vi "FindGit.vi"(8 "error in (no error)":errorcluster) -> (0 "error out":errorcluster, 2 "User Cancelled":bool, 3 "Git String":string)   [LabVIEW 2013]
uses:
  <vilib>/Utility/sysdir.llb/System Directory Type.ctl
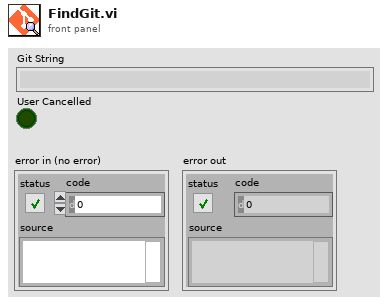
[diagram p1: front panel]
types:
  T1 = typedef "System Directory Type.ctl" = i32
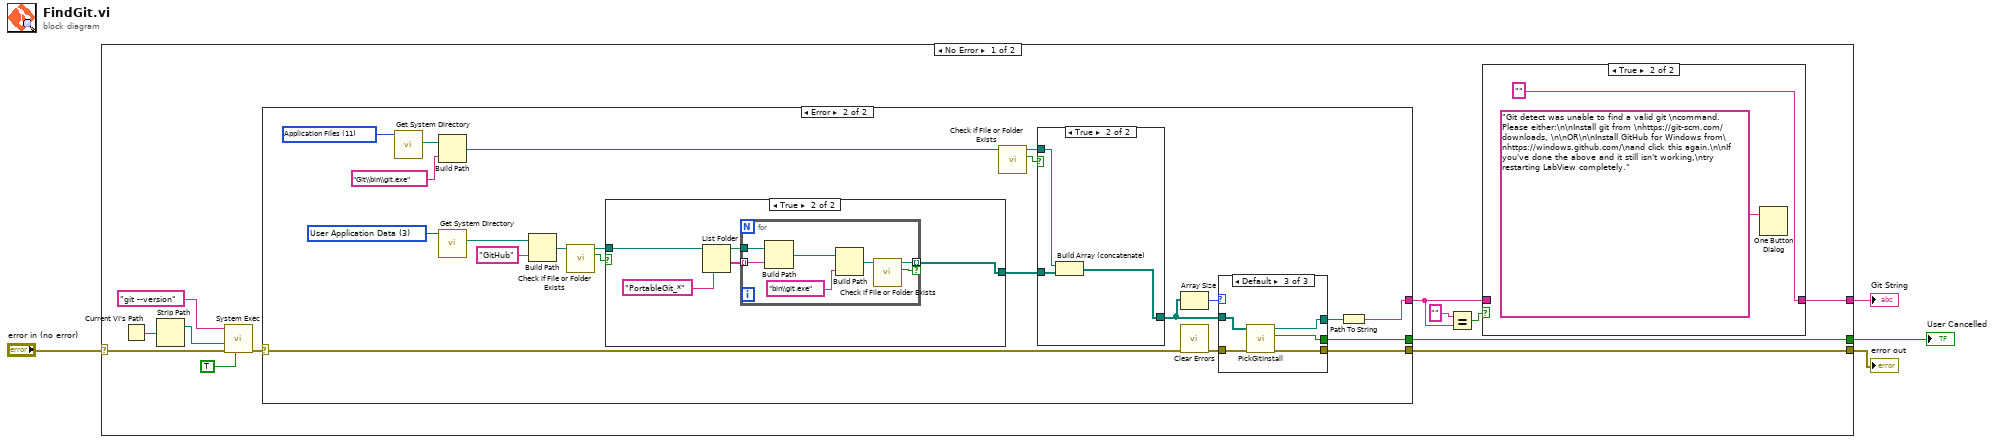
[diagram p0: block diagram]
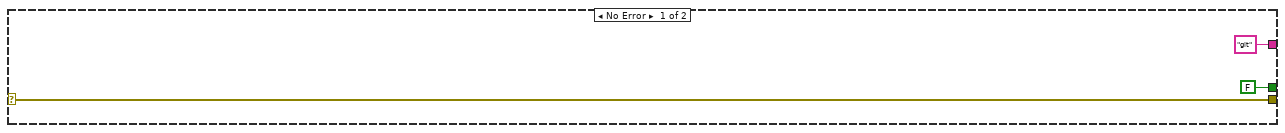
[diagram p3: hidden frame]
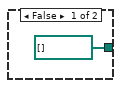
[diagram p4: hidden frame]
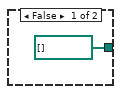
[diagram p5: hidden frame]
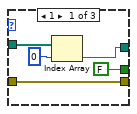
[diagram p6: hidden frame]
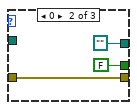
[diagram p7: hidden frame]
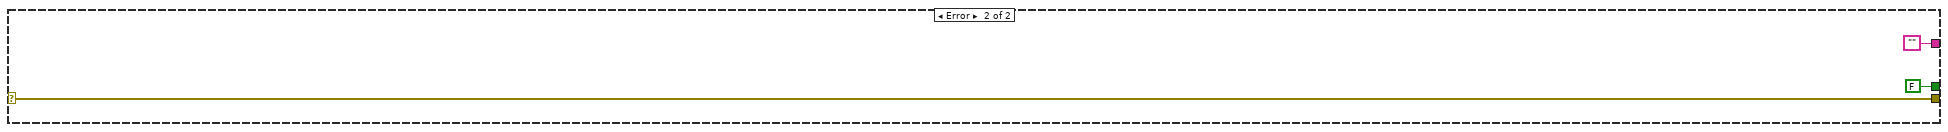
[diagram p8: hidden frame]
diagram:
  n1 = case shown="No Error" "error in (no error)" {
    selector: "error in (no error)" -> [w10 w76]
    tunnel: [w12 FALSE ("User Cancelled")] -> w4
    tunnel: [w6 ""] -> w3
    tunnel: [w9 w76] -> w2
    frame No Error {
      n2 = Current VI's Path() -> (path=w15:path)
      n3 = Strip Path(path=w15) -> (stripped path=w14:path)  [unwired: 1 out]
      n4 = call <vilib>:"System Exec.vi"("run minimized? (F)"=TRUE, "error in (no error)"=w10, "working directory"=w14, "command line"="git --version") -> ("error out"=w13:errorcluster)  [unwired: 4 in, 3 out]
      n5 = case shown="Error" w13 {
        selector: w13 -> [w20 w40]
        tunnel: [FALSE ("User Cancelled") w43] -> w12
        tunnel: ["git" w41] -> w5
        tunnel: [w20 w39] -> w9
        frame No Error {
        }
        frame Error {
          w27 = T1 11 items=["User Home"=0, "User Desktop"=1, "User Documents"=2, "User Application Data"=3, "User Preferences"=4, "User Temporary"=5, "Public Documents"=6, "Public Application Data"=7, "Public Preferences"=8, "Public Cache"=13, "System Core Libraries"=9, "System Installed Libraries"=10, "Application Files"=11, "Boot Volume Root"=12] ("system directory type")
          w38 = T1 3 items=["User Home"=0, "User Desktop"=1, "User Documents"=2, "User Application Data"=3, "User Preferences"=4, "User Temporary"=5, "Public Documents"=6, "Public Application Data"=7, "Public Preferences"=8, "Public Cache"=13, "System Core Libraries"=9, "System Installed Libraries"=10, "Application Files"=11, "Boot Volume Root"=12] ("system directory type")
          n6 = call <vilib>:"Get System Directory.vi"("system directory type"=w27) -> ("system directory"=w28:path)  [unwired: 10 in]
          n7 = Build Path(base path=w28, name or relative path="Git\\bin\\git.exe") -> (appended path=w30:path)
          n8 = call <vilib>:"Get System Directory.vi"("system directory type"=w38) -> ("system directory"=w36:path)  [unwired: 10 in]
          n9 = Build Path(base path=w36, name or relative path="GitHub") -> (appended path=w33:path)
          n10 = call <vilib>:"Check if File or Folder Exists.vi"("path"=w33) -> ("file or folder exists?"=w32:bool, "dup path"=w31:path)  [unwired: 8 in, 1 out]
          n11 = case shown="True" w32 {
            tunnel: [path[] [] w50] -> w24
            tunnel: w31 -> [_ w49]
            frame False {
            }
            frame True {
              n12 = List Folder(path=w49, pattern="PortableGit_*") -> (path out=w52:path, folder names=w51:string[])  [unwired: 2 in, 2 out]
              n13 = for {
                tunnel: w52 -> [w60]
                tunnel: w51 -> [w59] mode=indexing
                tunnel: [w55] -> w50 mode=indexing if=w54
                n14 = Build Path(base path=w60, name or relative path=w59) -> (appended path=w58:path)
                n15 = Build Path(base path=w58, name or relative path="bin\\git.exe") -> (appended path=w56:path)
                n16 = call <vilib>:"Check if File or Folder Exists.vi"("path"=w56) -> ("file or folder exists?"=w54:bool, "dup path"=w55:path)  [unwired: 8 in, 1 out]
              }
            }
          }
          n17 = call <vilib>:"Check if File or Folder Exists.vi"("path"=w30) -> ("file or folder exists?"=w26:bool, "dup path"=w25:path)  [unwired: 8 in, 1 out]
          n18 = case shown="True" w26 {
            tunnel: w25 -> [_ w47]
            tunnel: w24 -> [_ w46]
            tunnel: [path[] [] w45] -> w23
            frame False {
            }
            frame True {
              n19 = Build Array (concatenate)(w47, w46) -> (w45:path[])
            }
          }
          n20 = Array Size(array=w23) -> (size(s)=w37:i32)
          n21 = call <vilib>:"Clear Errors.vi"("error in (no error)"=w40) -> ("error out"=w35:errorcluster)  [unwired: 6 in]
          n22 = case shown="Default" w37 {
            tunnel: [w64 path "" w73] -> w42
            tunnel: w23 -> [w65 _ w72]
            tunnel: [FALSE FALSE ("User Cancelled") w71] -> w43
            tunnel: w35 -> [w62 w68 w70]
            tunnel: [w62 w68 w69] -> w39
            frame 1 {
              n23 = Index Array(array=w65, index=0) -> (element=w64:path)
            }
            frame 0 {
            }
            frame Default {
              n24 = call "PickGitInstall.vi"("error in (no error)"=w70, "Git Installs"=w72) -> ("error out"=w69:errorcluster, "User Cancelled"=w71:bool, "Git Path"=w73:path)  [unwired: 7 in]
            }
          }
          n25 = Path To String(path=w42) -> (string=w41:string)
        }
      }
      n26 = Equal?(x="", y=w5) -> (x = y?=w7:bool)
      n27 = case shown="True" w7 {
        tunnel: w5 -> [w17 _]
        tunnel: [w17 "" ("x")] -> w6
        frame False {
        }
        frame True {
          n28 = One Button Dialog(message="Git detect was unable to find a valid git \ncommand. Please either:\n\nInstall git from \nhttps://git-scm.com/downloads, \n\nOR\n\nInstall GitHub for Windows from\nhttps://windows.github.com/\nand click this again.\n\nIf you've done the above and it still isn't working,\ntry restarting LabView completely.") -> ()  [unwired: 1 in, 1 out]
        }
      }
    }
    frame Error {
    }
  }
  "User Cancelled" <- w4
  "Git String" <- w3
  "error out" <- w2
